vi "publish -- read -- num.vi"(8 "request event":refnum<user-event>, 9 "response in":refnum<user-event>) -> (1 "response out":refnum<user-event>, 3 "Numeric":dbl format="%#_13g")   [LabVIEW 2018]
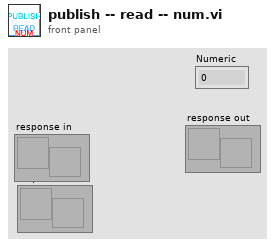
[diagram p1: front panel]
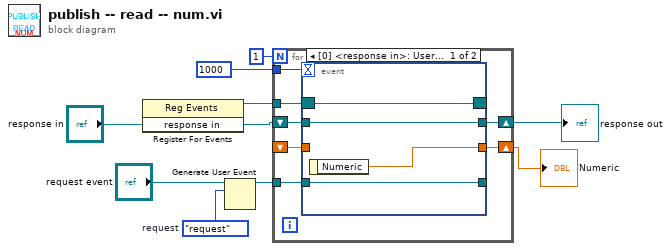
[diagram p0: block diagram]
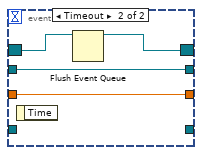
[diagram p2: hidden frame]
diagram:
  w9 = enum16{"request"}."request"  # request
  n1 = register-events("response in") -> (reference out=w6:refnum<event-registration>)  [unwired: 2 in, 1 out]
  n2 = Generate User Event(user event="request event", event data cluster=w9) -> (user event out=w7:refnum<user-event>)  [unwired: 2 in, 1 out]
  n3 = for {
    N: 1 -> [_]
    tunnel: w7 -> [w16]
    tunnel: w6 -> [w15]
    tunnel: 1000 -> [w14]
    shift-right: [w12] -> w3
    shift-left: "response in" -> [w13]
    shift-right: [w11] -> w2
    shift-left: _ -> [w10]
    n4 = event shown="[0] <response in>: User Event" {
      selector: w15 -> [w19 w24]
      dyn-events: [w19 w23] -> _
      timeout: w14 -> [_ _]
      tunnel: [w20 _] -> _
      tunnel: w16 -> [w20 _]
      tunnel: [w18 w22] -> w12
      tunnel: w13 -> [w18 w22]
      tunnel: [w17 w21] -> w11
      tunnel: w10 -> [_ w21]
      event User Event {
        n5 = event-data() -> ("Numeric"=w17:dbl)  [unwired: 1 in]
      }
      event Timeout {
        n6 = event-data() -> ()  [unwired: 1 in, 1 out]
        n7 = Flush Event Queue(0:w24) -> (8:w23:refnum<event-registration>)  [unwired: 5 in, 2 out]
      }
    }
  }
  "Numeric" <- w2
  "response out" <- w3
